vi "SPT-Initialize.vi"(0 "SPT In":T1, 11 "error in (no error)":errorcluster) -> (15 "error out":errorcluster)   [LabVIEW 2015]
uses:
  SPT-Data.ctl
  SPT-Properties.ctl
  SPT-Shape.ctl
  SPT-State.ctl
panel:
  out "SPT Out":T1
  in  "Fs (Hz)":dbl
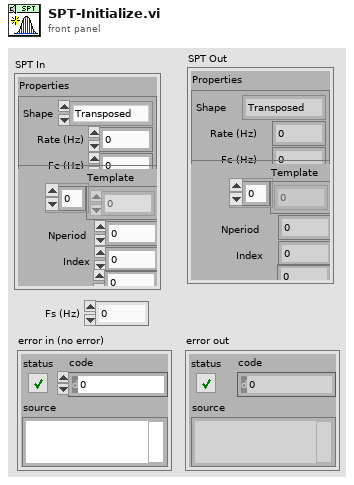
[diagram p1: front panel]
types:
  T1 = typedef "SPT-Data.ctl" = cluster{"Properties":T2, "State":T4}
  T2 = typedef "SPT-Properties.ctl" = cluster{"Shape":T3, "Rate (Hz)":dbl, "Fc (Hz)":dbl, "Width (ms)":dbl}
  T3 = typedef "SPT-Shape.ctl" = enum16{"Transposed", "Alpha", "Gabor"}
  T4 = typedef "SPT-State.ctl" = cluster{"Template":dbl[], "Nperiod":i32, "Index":i32, "Pulse Rate (Hz)":dbl, "Phase (cycles)":dbl, "Noff":i32}
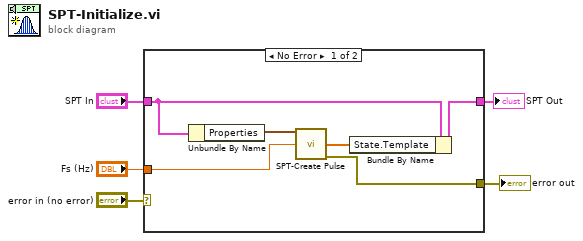
[diagram p0: block diagram]
diagram:
  n1 = case shown="No Error" "error in (no error)" {
    selector: "error in (no error)" -> [_ w13]
    tunnel: "SPT In" -> [w9 w12]
    tunnel: "Fs (Hz)" -> [w11 _]
    tunnel: [w7 w13] -> w2
    tunnel: [w6 w12] -> w1
    frame No Error {
      n2 = Unbundle By Name(w9) -> ("Properties"=w10:T2)
      n3 = call "SPT-Create Pulse.vi"("SPT.Properties"=w10, "Fs (Hz)"=w11) -> ("Pulse"=w8:dbl[], "error out"=w7:errorcluster)  [unwired: 12 in]
      n4 = Bundle By Name(cluster=w9, "State.Template"=w8) -> (w6:T1)
    }
    frame Error {
    }
  }
  "error out" <- w2
  "SPT Out" <- w1
